vi "SET_DEVICE_SET_DURATION_TO_GLOBAL.vi"(6 "DEVICE_SN":string, 9 "RANGE":string, 10 "DURATION":u16, 11 "USB_DEV":string) -> (2 "JSON string DEV":string, 3 "DEVICE? 2":bool)   [LabVIEW 2015]
uses:
  Share Data/uPower_kit.ctl
panel:
  in  "DEV_BUSY in":T1
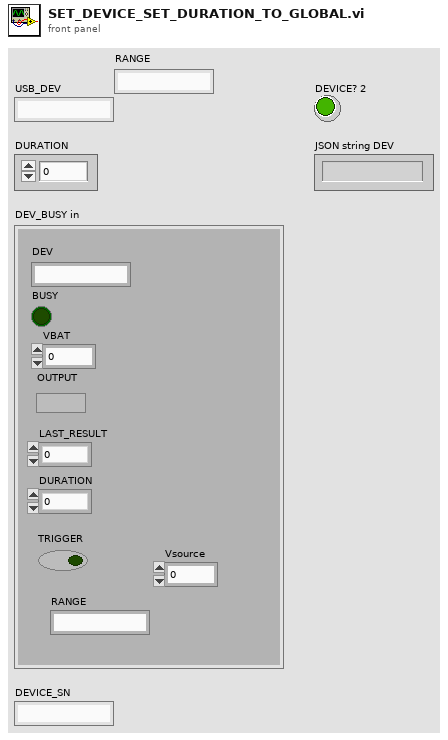
[diagram p1: front panel]
types:
  T1 = typedef "uPower_kit.ctl" = cluster{"DEV":string, "BUSY":bool, "VBAT":dbl, "OUTPUT":bool, "LAST_RESULT":dbl, "DURATION":u16, "TRIGGER":bool, "RANGE":string, "Vsource":dbl}
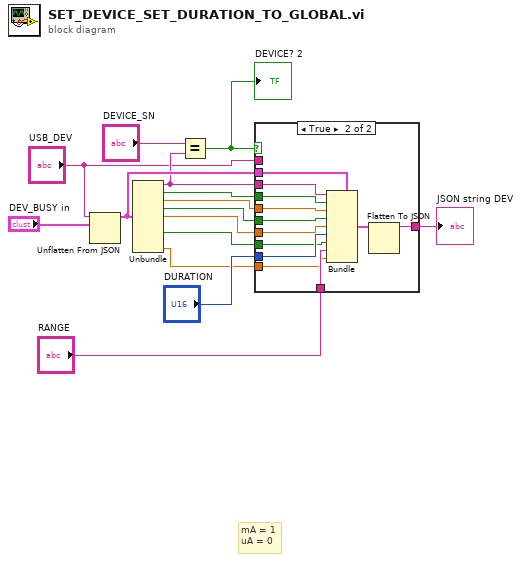
[diagram p0: block diagram]
diagram:
  # "mA = 1\nuA = 0"
  n1 = Unflatten From JSON(JSON string="USB_DEV", type and defaults="DEV_BUSY in") -> (value=w11:T1)  [unwired: 5 in, 1 out]
  n2 = Unbundle(w11) -> ("DEV"=w9:string, "BUSY"=w8:bool, "VBAT"=w7:dbl, "OUTPUT"=w6:bool, "LAST_RESULT"=w5:dbl, "TRIGGER"=w3:bool, "Vsource"=w1:dbl)  [unwired: 2 out]
  n3 = Equal?(x="DEVICE_SN", y=w9) -> (x = y?=w10:bool)
  "DEVICE? 2" <- w10
  n4 = case shown="True" w10 {
    tunnel: w11 -> [_ w28]
    tunnel: w9 -> [_ w27]
    tunnel: w8 -> [_ w26]
    tunnel: w7 -> [_ w22]
    tunnel: w6 -> [_ w21]
    tunnel: w5 -> [_ w25]
    tunnel: [w16 w23] -> w13
    tunnel: "USB_DEV" -> [w16 _]
    tunnel: "DURATION" -> [_ w20]
    tunnel: w3 -> [_ w19]
    tunnel: "RANGE" -> [_ w18]
    tunnel: w1 -> [_ w17]
    frame False {
    }
    frame True {
      n5 = Bundle(cluster=w28, "DEV"=w27, "BUSY"=w26, "VBAT"=w22, "OUTPUT"=w21, "LAST_RESULT"=w25, "DURATION"=w20, "TRIGGER"=w19, "RANGE"=w18, "Vsource"=w17) -> (w24:T1)
      n6 = Flatten To JSON(anything=w24) -> (JSON string=w23:string)  [unwired: 2 in, 1 out]
    }
  }
  "JSON string DEV" <- w13
